vi "Autonomous Independent.vi"() -> ()   [LabVIEW 2014]
doc: "This VI is called when autonomous begins, and will automatically be terminated when autonomous ends. You can carry out timed or sensor driven robot movement independently without needing to return to the caller."
panel:
  in  "Auto Mode":T1(ring)
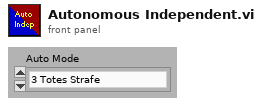
[diagram p1: front panel]
types:
  T1 = enum16{"3 Totes Strafe", "3 Totes Forward", "Move Forward Only", "Landfill"}
  T2 = enum16{"Move Forward", "Move Backward", "Strafe Right", "Strafe Left"}
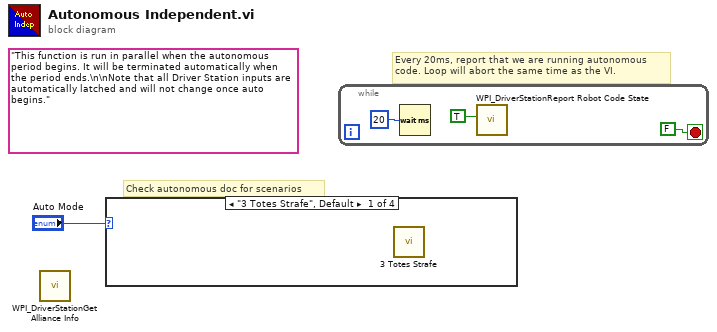
[diagram p0: block diagram]
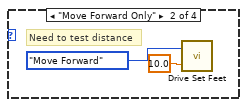
[diagram p2: hidden frame]
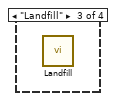
[diagram p3: hidden frame]
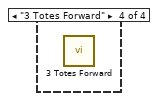
[diagram p4: hidden frame]
diagram:
  (unwired) "This function is run in parallel when the autonomous period begins. It will be terminated automatically when the period ends.\n\nNote that all Driver Station inputs are automatically latched and will not change once auto begins."
  # "Check autonomous doc for scenarios"
  # "Every 20ms, report that we are running autonomous\ncode. Loop will abort the same time as the VI."
  n1 = call <vilib>:"WPI_DriverStationGet Alliance Info.vi"() -> ()  [unwired: 12 out]
  n2 = case shown="\"3 Totes Strafe\", Default" "Auto Mode" {
    frame "3 Totes Strafe", Default {
      n3 = call "3 Totes Strafe.vi"() -> ()  [unwired: 12 in]
    }
    frame "Move Forward Only" {
      # "Need to test distance"
      n4 = call "Drive Set Feet.vi"("Feet"=10.0, "Direction"=T2."Move Forward") -> ()  [unwired: 1 out]
    }
    frame "Landfill" {
      n5 = call "Landfill.vi"() -> ()  [unwired: 12 in]
    }
    frame "3 Totes Forward" {
      n6 = call "3 Totes Forward.vi"() -> ()  [unwired: 12 in]
    }
  }
  n7 = while {
    stop <- FALSE stop-if-true
    n8 = Wait (ms)(milliseconds to wait=u32 20) -> ()  [unwired: 1 out]
    n9 = call <vilib>:"WPI_DriverStationReport Robot Code State.vi"("Autonomous"=TRUE) -> ()  [unwired: 10 in, 1 out]
  }
